vi "DAQmx Read (Power 1D Wfm NChan NSamp).vi"(0 "task/channels in":refnum<k21>, 7 "number of samples per channel":i32=-1, 9 "timeout":dbl=10.0 format="%0.2f", 11 "error in":errorcluster) -> (4 "task out":refnum<k21>, 6 "voltage":waveform(dbl)[](array[waveform]), 8 "current":waveform(dbl)[](array[waveform]), 15 "error out":errorcluster)   [LabVIEW 2024]
doc: "Reads one or more waveforms that contains one or more floating-point samples from a task that contains one or more power channels."
uses:
  nilvaiu.dll
panel:
  # "channel"
  # "channel"
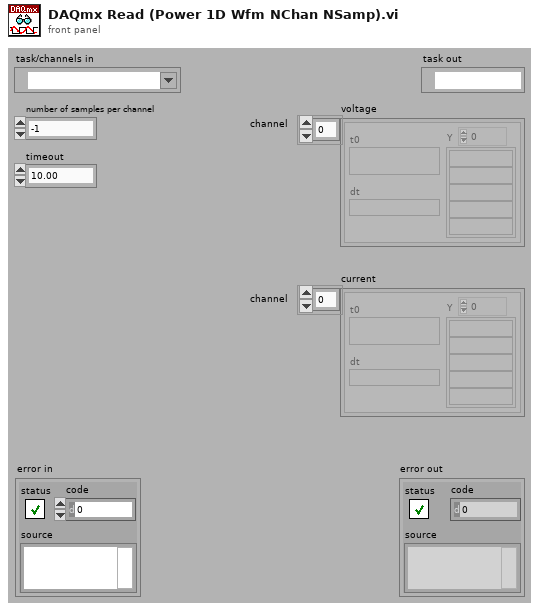
[diagram p1: front panel]
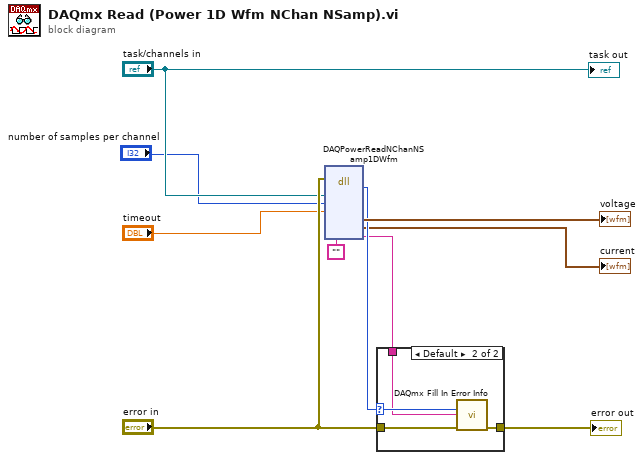
[diagram p0: block diagram]
diagram:
  n1 = dll-call lib="nilvaiu.*" fn="DAQPowerReadNChanNSamp1DWfm"(error in="error in", "taskID"="task/channels in", "samplesPerCHannel"="number of samples per channel", "timeout"="timeout", "extendedErrorInfo"="") -> ("return type"=w4:i32, "voltage"=→"voltage":waveform(dbl)[], "current"=→"current":waveform(dbl)[], "extendedErrorInfo"=w2:string)  [unwired: 4 in, 5 out]
  n2 = case shown="Default" w4 {
    selector: w4 -> [_ w13]
    tunnel: "error in" -> [w11 w15]
    tunnel: [w11 w14] -> w9
    tunnel: w2 -> [_ w12]
    frame 0 {
    }
    frame Default {
      n3 = call "DAQmx Fill In Error Info.vi"("status code"=w13, "extended error info"=w12, "error in"=w15) -> ("error out"=w14:errorcluster)  [unwired: 1 in, 11 out]
    }
  }
  "error out" <- w9
  "task out" <- "task/channels in"
